vi "Update square wave channel.vi"(8 "Error In":errorcluster, 9 "Value":dbl min=0.0 max=204.8000030517578 step=0.012500000186264515 format="%#_g V", 10 "Channel":u8 max=31 step=1, 11 "Arduino Port":refnum<visa-resource-name>) -> (0 "Error Out":errorcluster, 3 "Arduino Port out":refnum<visa-resource-name>)   [LabVIEW 2016]
doc: "Perform an update of the voltage output of the input channel of AD5535. The max speed of this operation is 1-2ms"
uses:
  Typedef/AD5535 - Command.ctl
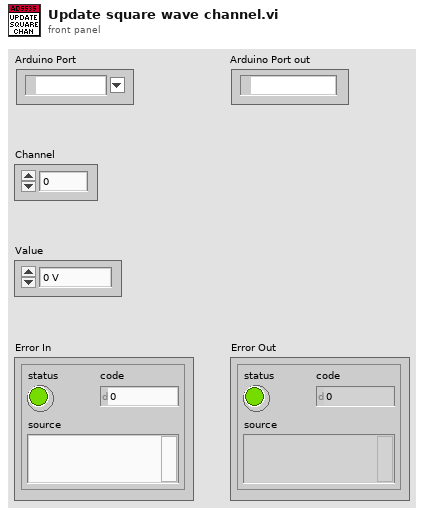
[diagram p1: front panel]
types:
  T1 = typedef "AD5535 - Command.ctl" = enum16{"None", "Start", "Stop", "Load Array", "Update channel", "Update frequency", "Prova"}
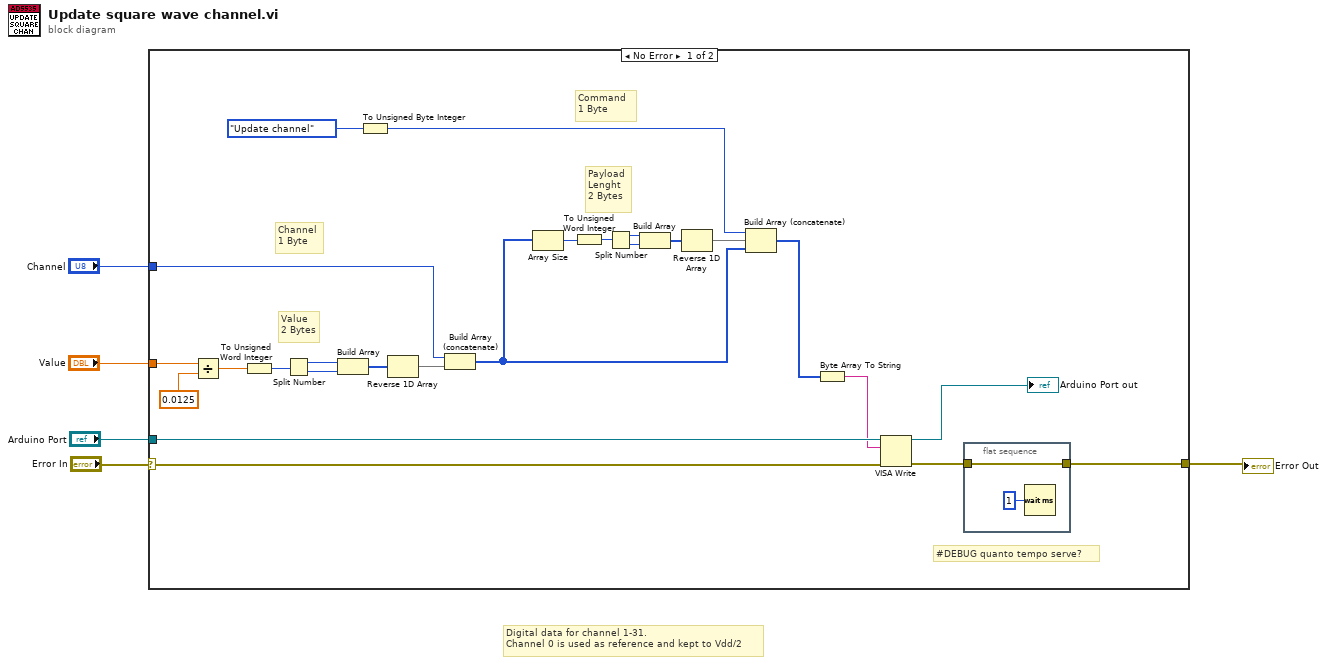
[diagram p0: block diagram]
diagram:
  # "Digital data for channel 1-31.\nChannel 0 is used as reference and kept to Vdd/2"
  n1 = case shown="No Error" "Error In" {
    selector: "Error In" -> [w29 w33]
    tunnel: [w26 w33] -> w4
    tunnel: "Arduino Port" -> [w30 _]
    tunnel: "Channel" -> [w7 _]
    tunnel: "Value" -> [w11 _]
    frame No Error {
      # "Value\n2 Bytes"
      # "Channel\n1 Byte"
      # "Command\n1 Byte"
      # "Payload\nLenght\n2 Bytes"
      # "#DEBUG quanto tempo serve?"
      n2 = Divide(x=w11, y=0.0125) -> (x/y=w13:dbl)
      n3 = To Unsigned Word Integer(number=w13) -> (unsigned 16bit integer=w14:u16)
      n4 = Split Number(x=w14) -> (hi(x)=w15:u8, lo(x)=w16:u8)
      n5 = Build Array(w15, w16) -> (w17:u8[])
      n6 = To Unsigned Byte Integer(number=AD5535_-_Command."Update channel" ("AD5535 - Command")) -> (unsigned 8bit integer=w24:u8)
      n7 = Reverse 1D Array(array=w17) -> (reversed array=w8:u8[])
      n8 = Build Array (concatenate)(w7, w8) -> (w6:u8[])
      n9 = Array Size(array=w6) -> (size(s)=w19:i32)
      n10 = To Unsigned Word Integer(number=w19) -> (unsigned 16bit integer=w20:u16)
      n11 = Split Number(x=w20) -> (hi(x)=w21:u8, lo(x)=w22:u8)
      n12 = Build Array(w21, w22) -> (w23:u8[])
      n13 = Reverse 1D Array(array=w23) -> (reversed array=w18:u8[])
      n14 = Build Array (concatenate)(w24, w18, w6) -> (w10:u8[])
      n15 = Byte Array To String(unsigned byte array=w10) -> (string=w9:string)
      n16 = VISA Write(VISA resource name=w30, write buffer=w9, error in (no error)=w29) -> (VISA resource name out=→"Arduino Port out":refnum<visa-resource-name>, error out=w27:errorcluster)  [unwired: 1 out]
      n17 = flat-sequence {
        tunnel: w27 -> [w32]
        tunnel: [w32] -> w26
        frame #0 {
          n18 = Wait (ms)(milliseconds to wait=u32 1) -> ()  [unwired: 1 out]
        }
      }
    }
    frame Error {
    }
  }
  "Error Out" <- w4
